vi "SortCalibrationPoints.vi"(1 "Array in":i32[][](array[numeric])) -> (0 "Array out":i32[][](array[numeric]))   [LabVIEW 2017]
panel:
  out "X3":i32[](array[numeric])
  out "X1":i32[](array[numeric])
  out "X4":i32[](array[numeric])
  out "X2":i32[](array[numeric])
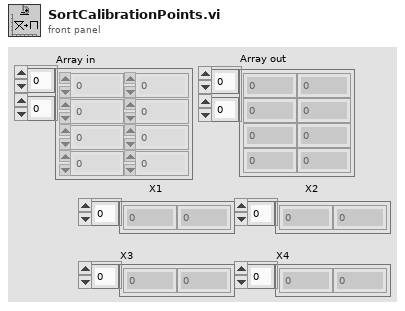
[diagram p1: front panel]
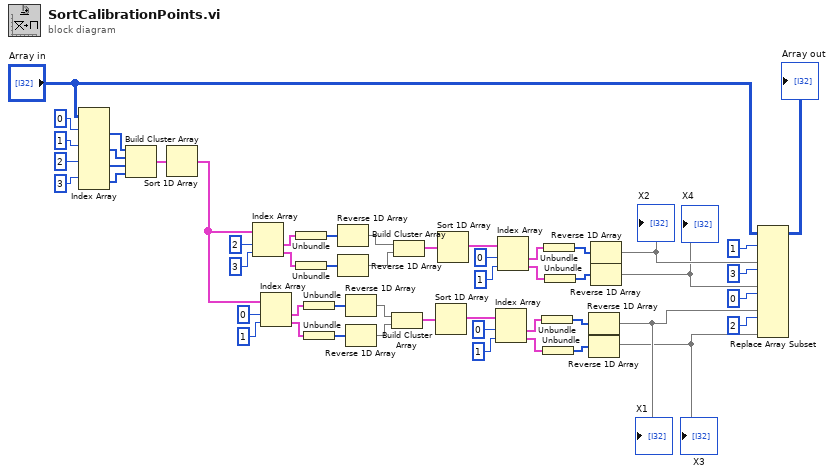
[diagram p0: block diagram]
diagram:
  n1 = Index Array(array="Array in", index (row) #1=0 ("index (row)"), index (row) #2=1 ("index (row)"), index (row) #3=2 ("index (row)"), index (row) #4=3 ("index (row)")) -> (element #1=w44:i32[], element #2=w45:i32[], element #3=w46:i32[], element #4=w47:i32[])  [unwired: 4 in]
  n2 = Build Cluster Array(w44, w45, w46, w47) -> (w43:cluster{"Array in":i32[]}[])
  n3 = Sort 1D Array(array=w43) -> (sorted array=w23:cluster{"Array in":i32[]}[])
  n4 = Index Array(array=w23, index #1=2 ("index"), index #2=3 ("index")) -> (element #1=w49:cluster{"Array in":i32[]}, element #2=w50:cluster{"Array in":i32[]})
  n5 = Index Array(array=w23, index #1=0 ("index"), index #2=1 ("index")) -> (element #1=w35:cluster{"Array in":i32[]}, element #2=w34:cluster{"Array in":i32[]})
  n6 = Unbundle(w49) -> ("Array in"=w52:i32[])
  n7 = Unbundle(w50) -> ("Array in"=w51:i32[])
  n8 = Unbundle(w35) -> ("Array in"=w32:i32[])
  n9 = Unbundle(w34) -> ("Array in"=w33:i32[])
  n10 = Reverse 1D Array(array=w52) -> (reversed array=w4:i32[])
  n11 = Reverse 1D Array(array=w51) -> (reversed array=w3:i32[])
  n12 = Reverse 1D Array(array=w32) -> (reversed array=w22:i32[])
  n13 = Reverse 1D Array(array=w33) -> (reversed array=w21:i32[])
  n14 = Build Cluster Array(w22, w21) -> (w20:cluster{i32[]}[])
  n15 = Build Cluster Array(w4, w3) -> (w5:cluster{i32[]}[])
  n16 = Sort 1D Array(array=w20) -> (sorted array=w19:cluster{i32[]}[])
  n17 = Sort 1D Array(array=w5) -> (sorted array=w6:cluster{i32[]}[])
  n18 = Index Array(array=w19, index #1=0 ("index"), index #2=1 ("index")) -> (element #1=w15:cluster{i32[]}, element #2=w16:cluster{i32[]})
  n19 = Index Array(array=w6, index #1=0 ("index"), index #2=1 ("index")) -> (element #1=w10:cluster{i32[]}, element #2=w9:cluster{i32[]})
  n20 = Unbundle(w15) -> (w14:i32[])
  n21 = Unbundle(w16) -> (w13:i32[])
  n22 = Unbundle(w10) -> (w2:i32[])
  n23 = Unbundle(w9) -> (w1:i32[])
  n24 = Reverse 1D Array(array=w14) -> (reversed array=w12:i32[])
  "X1" <- w12
  n25 = Reverse 1D Array(array=w13) -> (reversed array=w11:i32[])
  "X3" <- w11
  n26 = Reverse 1D Array(array=w2) -> (reversed array=w27:i32[])
  "X2" <- w27
  n27 = Reverse 1D Array(array=w1) -> (reversed array=w26:i32[])
  "X4" <- w26
  n28 = Replace Array Subset(array="Array in", new element #1=w27, index (row) #1=1 ("index (row)"), new element #2=w26, index (row) #2=3 ("index (row)"), new element #3=w12, index (row) #3=0 ("index (row)"), new element #4=w11, index (row) #4=2 ("index (row)")) -> (→"Array out":i32[][])  [unwired: 4 in]
